vi "AIM664 Receive Continuous Capture.vi"() -> ()   [LabVIEW 2020]
uses:
  AIM664LV.lvlib
panel:
  out "QueueIdOut 2":u32
  out "GlobMonSize 2":u32=2153143691
  out "QueueIdOut":u32
  out "GlobMonSize":u32=2153143691
  in  "Strobe":u32(ring) items=["FDX_MON_STROBE_DIS", "FDX_MON_STROBE_STOP", "FDX_MON_STROBE_START"]
  in  "TriggerPosition":u32
  in  "CaptureMode":u32(ring)=1 items=["FDX_MON_SINGLE ", "FDX_MON_CONTINUOUS", "FDX_MON_SELECTIVE", "FDX_MON_RECORDING", "FDX_MON_REROS", "FDX_MON_HMU"]
  out "QueueStatus":T1 {"QueueStatus" items=["FDX_MON_STAT_EMPTY", "FDX_MON_STAT_ FILLED", "FDX_MON_STAT_ FULL", "FDX_MON_STAT_ OVERFLOW", "FDX_MON_STAT_ ERROR"]}
  out "GlobalStat Out":T2
  in  "Control":u32(ring) items=["FDX_RX_GS_RES_NO_CNT", "FDX_RX_GS_RES_ALL_CNT", "FDX_RX_GS_RES_ERR_CNT"]
  in  "PortMap":u32=1
  out "PortInitOut":T3 {"PortConfig" items=["FDX_SINGLE", "FDX_REDUNDANT"]}
  out "ResourceInfo 2":T4 {"PortMode" items=[" FDX_SINGLE", "FDX_REDUNDANT"]}
  out "ResourceInfo":T4 {"PortMode" items=[" FDX_SINGLE", "FDX_REDUNDANT"]}
  in  "Input Cluster 2":T5={"QueueCtrl"=1, "QueueId"=0, "RecordingFileName"="", "MaxFileSize"=0} {"QueueCtrl" items=["FDX_MON_QUEUE_CREATE", "FDX_MON_QUEUE_DELETE"]}
  in  "Stopp":bool
  out "Output Cluste":T6={"EntryRead"=0, "BytesRead"=0, "Synchronized"=0, "ReadBuffer"=[0, 0, 0, 0, 0, 0, 0, 0, 0, 0, 0, 0, 0, 0, 0, 0, 60, 0, 0, 0, 64, 64, 0, 48, 84, 0, 128, 0, 104, 8, 0, 0, 33, 75, 42, 162, 3, 0, 0, 0, 0, 60, 2, 0, 0, 1, 33, 32, 8, 0, 69, 0, 0, 45, 0, 0, 64, 0, 1, 17, 109, 162, 10, 1, 33, 1, 224, 224, 0, 60, 0, 24, 0, 23, 0, 25, 0, 0, 65, 66, 67, 68, 69, 70, 71, 72, 73, 74, 75, 76, 77, 78, 79, 80, 81, 84, 0, 5, 0, 5, 0, 5, 0, 5, 0, 5, 0, 5, 0, 5, 0, 5, 0, 5, 0, 5, 0, 5, 0, 5, 0, 5, 0, 5, 0, 5, 0, 5, 0, 0, 0, 0, 0, 0, 0, 0, 0, 0, 0, 0, 0, 0, 0, 0, 0, 0, 0, 0, 0, 0, 0, 0, 0, 0, 0, 0, 0, 0, 0, 0, 0, 0, 0, 0, 0, 0, 0, 0, 0, 0, 0, 0, 0, 0, 0, 0, 0, 0, 0, 0, 0, 0, 0, 0, 0, 0, 0, 0, 0, 0, 0, 0, 0, 0, 0, 0, 0, 0, 0, 0, 0, 0, 0, 0, 0, 0, 0, 0, 0, 0, 0, 0, 0, 0, 0, 0, 0, 0, 0, 0, 0, 0, 0, 0, 0, 0, 0, 0, 0, 0, 0, 0, 0, 0, 0, 0, 0, 0, 0, 0, 0, 0, 0, 0, 0, 0, 0, 0, 0, 0, 0, 0, 0, 0, 0, 0, 0, 0, 0, 0, 0, 0, 0, 0, 0, 0, 0, 0, 0, 0, 0, 0, 0, 0, 0, 0, 0, 0, 0, 0, 0, 0, 0, 0, 0, 0, 0, 0, 0, 0, 0, 0, 0, 0, 0, 0, 0, 0, 0, 0, 0, 0, 0, 0, 0, 0, 0, 0, 0, 0, 0, 0, 0, 0, 0, 0, 0, 0, 0, 0, 0, 0, 0, 0, 0, 0, 0, 0, 0, 0, 0, 0, 0, 0, 0, 0, 0, 0, 0, 0, 0, 0, 0, 0, 0, 0, 0, 0, 0, 0, 0, 0, 0, 0, 0, 0, 0, 0, 0, 0, 0, 0, 0, 0, 0, 0, 0, 0, 0, 0, 0, 0, 0, 0, 0, 0, 0, 0, 0, 0, 0, 0, 0, 0, 0, 0, 0, 0, 0, 0, 0, 0, 0, 0, 0, 0, 0, 0, 0, 0, 0, 0, 0, 0, 0, 0, 0, 0, 0, 0, 0, 0, 0, 0, 0, 0, 0, 0, 0, 0, 0, 0, 0, 0, 0, 0, 0, 0, 0, 0, 0, 0, 0, 0, 0, 0, 0, 0, 0, 0, 0, 0, 0, 0, 0, 0, 0, 0, 0, 0, 0, 0, 0, 0, 0, 0, 0, 0, 0, 0, 0, 0, 0, 0, 0, 0, 0, 0, 0, 0, 0, 0, 0, 0, 0, 0, 0, 0, 0, 0, 0, 0, 0, 0, 0, 0, 0, 0, 0, 0, 0, 0, 0, 0, 0, 0, 0, 0, 0, 0, 0, 0, 0, 0, 0, 0, 0, 0, 0, 0, 0, 0, 0, 0, 0, 0, 0, 0, 0, 0, 0, 0, 0, 0, 0, 0, 0, 0, 0, 0, 0, 0, 0, 0, 0, 0, 0, 0, 0, 0, 0, 0, 0, 0, 0, 0, 0, 0, 0, 0, 0, 0, 0, 0, 0, 0, 0, 0, 0, 0, 0, 0, 0, 0, 0, 0, 0, 0, 0, 0, 0, 0, 0, 0, 0, 0, 0, 0, 0, 0, 0, 0, 0, 0, 0, 0, 0, 0, 0, 0, 0, 0, 0, 0, 0, 0, 0, 0, 0, 0, 0, 0, 0, 0, 0, 0, 0, 0, 0, 0, 0, 0, 0, 0, 0, 0, 0, 0, 0, 0, 0, 0, 0, 0, 0, 0, 0, 0, 0, 0, 0, 0, 0, 0, 0, 0, 0, 0, 0, 0, 0, 0, 0, 0, 0, 0, 0, 0, 0, 0, 0, 0, 0, 0, 0, 0, 0, 0, 0, 0, 0, 0, 0, 0, 0, 0, 0, 0, 0, 0, 0, 0, 0, 0, 0, 0, 0, 0, 0, 0, 0, 0, 0, 0, 0, 0, 0, 0, 0, 0, 0, 0, 0, 0, 0, 0, 0, 0, 0, 0, 0, 0, 0, 0, 0, 0, 0, 0, 0, 0, 0, 0, 0, 0, 0, 0, 0, 0, 0, 0, 0, 0, 0, 0, 0, 0, 0, 0, 0, 0, 0, 0, 0, 0, 0, 0, 0, 0, 0, 0, 0, 0, 0, 0, 0, 0, 0, 0, 0, 0, 0, 0, 0, 0, 0, 0, 0, 0, 0, 0, 0, 0, 0, 0, 0, 0, 0, 0, 0, 0, 0, 0, 0, 0, 0, 0, 0, 0, 0, 0, 0, 0, 0, 0, 0, 0, 0, 0, 0, 0, 0, 0, 0, 0, 0, 0, 0, 0, 0, 0, 0, 0, 0, 0, 0, 0, 0, 0, 0, 0, 0, 0, 0, 0, 0, 0, 0, 0, 0, 0, 0, 0, 0, 0, 0, 0, 0, 0, 0, 0, 0, 0, 0, 0, 0, 0, 0, 0, 0, 0, 0, 0, 0, 0, 0, 0, 0, 0, 0, 0, 0, 0, 0, 0, 0, 0, 0, 0, 0, 0, 0, 0, 0, 0, 0, 0, 0, 0, 0, 0, 0, 0, 0, 0, 0, 0, 0, 0, 0, 0, 0, 0, 0, 0, 0, 0, 0, 0, 0, 0, 0, 0, 0, 0, 0, 0, 0, 0, 0, 0, 0, 0, 0, 0, 0, 0, 0, 0, 0, 0, 0, 0, 0, 0, 0, 0, 0, 0, 0, 0, 0, 0, 0, 0, 0, 0, 0, 0, 0, 0, 0, 0, 0, 0, 0, 0, 0, 0, 0, 0, 0, 0, 0, 0, 0, 0, 0, 0, 0, 0, 0, 0, 0, 0, 0, 0, 0, 0, 0, 0, 0, 0, 0, 0, 0, 0, 0, 0, 0, 0, 0, 0, 0, 0, 0, 0, 0, 0, 0, 0, 0, 0, 0, 0, 0, 0, 0, 0, 0, 0, 0, 0, 0, 0, 0, 0, 0, 0, 0, 0, 0, 0, 0, 0, 0, 0, 0, 0, 0, 0, 0, 0, 0, 0, 0, 0, 0, 0, 0, 0, 0, 0, 0, 0, 0, 0, 0, 0, 0, 0, 0, 0, 0, 0, 0, 0, 0, 0, 0, 0, 0, 0, 0, 0, 0, 0, 0, 0, 0, 0, 0, 0, 0, 0, 0, 0, 0, 0, 0, 0, 0, 0, 0, 0, 0, 0, 0, 0, 0, 0, 0, 0, 0, 0, 0, 0, 0, 0, 0, 0, 0, 0, 0, 0, 0, 0, 0, 0, 0, 0, 0, 0, 0, 0, 0, 0, 0, 0, 0, 0, 0, 0, 0, 0, 0, 0, 0, 0, 0, 0, 0, 0, 0, 0, 0, 0, 0, 0, 0, 0, 0, 0, 0, 0, 0, 0, 0, 0, 0, 0, 0, 0, 0, 0, 0, 0, 0, 0, 0, 0, 0, 0, 0, 0, 0, 0, 0, 0, 0, 0, 0, 0, 0, 0, 0, 0, 0, 0, 0, 0, 0, 0, 0, 0, 0, 0, 0, 0, 0, 0, 0, 0, 0, 0, 0, 0, 0, 0, 0, 0, 0, 0, 0, 0, 0, 0, 0, 0, 0, 0, 0, 0, 0, 0, 0, 0, 0, 0, 0, 0, 0, 0, 0, 0, 0, 0, 0, 0, 0, 0, 0, 0, 0, 0, 0, 0, 0, 0, 0, 0, 0, 0, 0, 0, 0, 0, 0, 0, 0, 0, 0, 0, 0, 0, 0, 0, 0, 0, 0, 0, 0, 0, 0, 0, 0, 0, 0, 0, 0, 0, 0, 0, 0, 0, 0, 0, 0, 0, 0, 0, 0, 0, 0, 0, 0, 0, 0, 0, 0, 0, 0, 0, 0, 0, 0, 0, 0, 0, 0, 0, 0, 0, 0, 0, 0, 0, 0, 0, 0, 0, 0, 0, 0, 0, 0, 0, 0, 0, 0, 0, 0, 0, 0, 0, 0, 0, 0, 0, 0, 0, 0, 0, 0, 0, 0, 0, 0, 0, 0, 0, 0, 0, 0, 0, 0, 0, 0, 0, 0, 0, 0, 0, 0, 0, 0, 0, 0, 0, 0, 0, 0, 0, 0, 0, 0, 0, 0, 0, 0, 0, 0, 0, 0, 0, 0, 0, 0, 0, 0, 0, 0, 0, 0, 0, 0, 0, 0, 0, 0, 0, 0, 0, 0, 0, 0, 0, 0, 0, 0, 0, 0, 0, 0, 0, 0, 0, 0, 0, 0, 0, 0, 0, 0, 0, 0, 0, 0, 0, 0, 0, 0, 0, 0, 0, 0, 0, 0, 0, 0, 0, 0, 0, 0, 0, 0, 0, 0, 0, 0, 0, 0, 0, 0, 0, 0, 0, 0, 0, 0, 0, 0, 0, 0, 0, 0, 0, 0, 0, 0, 0, 0, 0, 0, 0, 0, 0, 0, 0, 0, 0, 0, 0, 0, 0, 0, 0, 0, 0, 0, 0, 0, 0, 0, 0, 0, 0, 0, 0, 0, 0, 0, 0, 0, 0, 0, 0, 0, 0, 0, 0, 0, 0, 0, 0, 0, 0, 0, 0, 0, 0, 0, 0, 0, 0, 0, 0, 0, 0, 0, 0, 0, 0, 0, 0, 0, 0, 0, 0, 0, 0, 0, 0, 0, 0, 0, 0, 0, 0, 0, 0, 0, 0, 0, 0, 0, 0, 0, 0, 0, 0, 0, 0, 0, 0, 0, 0, 0, 0, 0, 0, 0, 0, 0, 0, 0, 0, 0, 0, 0, 0, 0, 0, 0, 0, 0, 0, 0, 0, 0, 0, 0, 0, 0, 0, 0, 0, 0, 0, 0, 0, 0, 0, 0, 0, 0, 0, 0, 0, 0, 0, 0, 0, 0, 0, 0, 0, 0, 0, 0, 0, 0, 0, 0, 0, 0, 0, 0, 0, 0, 0]} {"ReadBuffer" format="%x"}
  in  "Input Cluster":T7={"QueueId"=0, "EntryCount"=1, "ReadQualifier"=0, "MaxReadBytes"=1600} {"ReadQualifier" items=["FDX_MON_READ_FULL", "FDX_MON_READ_HEADER", "FDX_MON_READ_DATA"]}
  in  "Input Cluster":T5 {"QueueCtrl" items=["FDX_MON_QUEUE_CREATE", "FDX_MON_QUEUE_DELETE"]}
  in  "Input Cluster":T8={"ReceiveMode"=0, "DefaultPayloadMode"=0, "DefaultCronoMode"=1, "GlbMonBufferSizeIn"=0, "RerosDefaultOutputPortmap"=0} {"DefaultCronoMode" items=["cFDX_RX_DEFAULT_ENA_CNT", "FDX_RX_DEFAULT_MON_ENA_ALL", "FDX_RX_DEFAULT_MON_ENA_GOOD"]; "DefaultPayloadMode" items=["FDX_PAYLOAD_FULL", "FDX_PAYLOAD_IP_EXT", "FDX_PAYLOAD_IP", "FDX_PAYLOAD_MAC"]; "ReceiveMode" items=["FDX_RX_CHRONO", "FDX_RX_VL"]}
  out "GlbMonBufferSizeOut":u32
  in  "Input Cluster":T9={"SrvName"="local", "ClHostName"="local", "ClUser"="Brett", "ClApplication"="Test", "ClApplicationVersion"="V01.00", "ResourceID"=2, "Privileges"=4294967295} {"Privileges" items=["PRIVILEGES_ADMIN"=4294967295]}
  in  "Input Cluster":T9={"SrvName"="local", "ClHostName"="local", "ClUser"="Brett", "ClApplication"="Test", "ClApplicationVersion"="V01.00", "ResourceID"=1, "Privileges"=4294967295} {"Privileges" items=["PRIVILEGES_ADMIN"=4294967295]}
  in  "Input Cluster":T10={"SrvName"="local", "ResourceID"=1, "ResourceType"=0} {"ResourceType" items=["Board", "Port"]}
  out "Output Cluster 2":T11={"ResourceID"=0, "ResourceType"=0, "ResourceInfo"="0", "StructId"=0}
  in  "ServerRElement":u32=1
  in  "Input Cluster":T10={"SrvName"="local", "ResourceID"=2, "ResourceType"=1} {"ResourceType" items=["Board", "Port"]}
  out "Output Cluster":T11={"ResourceID"=0, "ResourceType"=0, "ResourceInfo"="0", "StructId"=0}
  in  "ServerRElement":u32=2
  out "NuOfResources":u32
  in  "SrvName":string="local"
  out "NuOfServers":u32=1
  # "ARINC 664 Receive Continuous Capture"
  # "Overview: Configure the board for Continuous Capture.\nRequirement: At least one AIM ARINC-664 board with installed AIM ARINC 664 BSP.\nRestrictions: None.\nInstruction:\n1. Run the VI.\n2. Verify the results in the indicators."
  # "Rx Port"
  # "Board"
  # "Rx Port"
  # "Board"
  # "FdxInitCvi"
  # "FdxLogoutCvi"
  # "CountServerResourcesCvi"
  # "GetServerResourcesCvi"
  # "QueryServerResourceCvi"
  # "FdxLoginCvi"
  # "FdxLogoutCvi"
  # "GetServerResourcesCvi"
  # "QueryServerResourceCvi"
  # "FdxRxModeControlCvi"
  # "FdxRxMonCaptureControlCvi"
  # "FdxLoginCvi"
  # "FdxCmdMonQueueControl"
  # "FdxRxControlCvi"
  # "FdxCmdMonQueueControl"
  # "FdxCmdRxPortInitCvi"
  # "FdxMonQueueStatusCvi"
  # "FdxCmdMonQueueReadCvi"
  # "FdxCmdRxGlblStatCvi"
  # "FdxRxControlCvi"
  # "Input"
  # "Input"
  # "Input"
  # "Input"
  # "Input"
  # "Input"
  # "Input"
  # "Input"
  # "Input"
  # "Output"
  # "Input"
  # "Input"
  # "Input"
  # "Input"
  # "Input"
  # "Input"
  # "Output"
  # "Output"
  # "Output"
  # "Output"
  # "Output"
  # "Output"
  # "Output"
  # "Output"
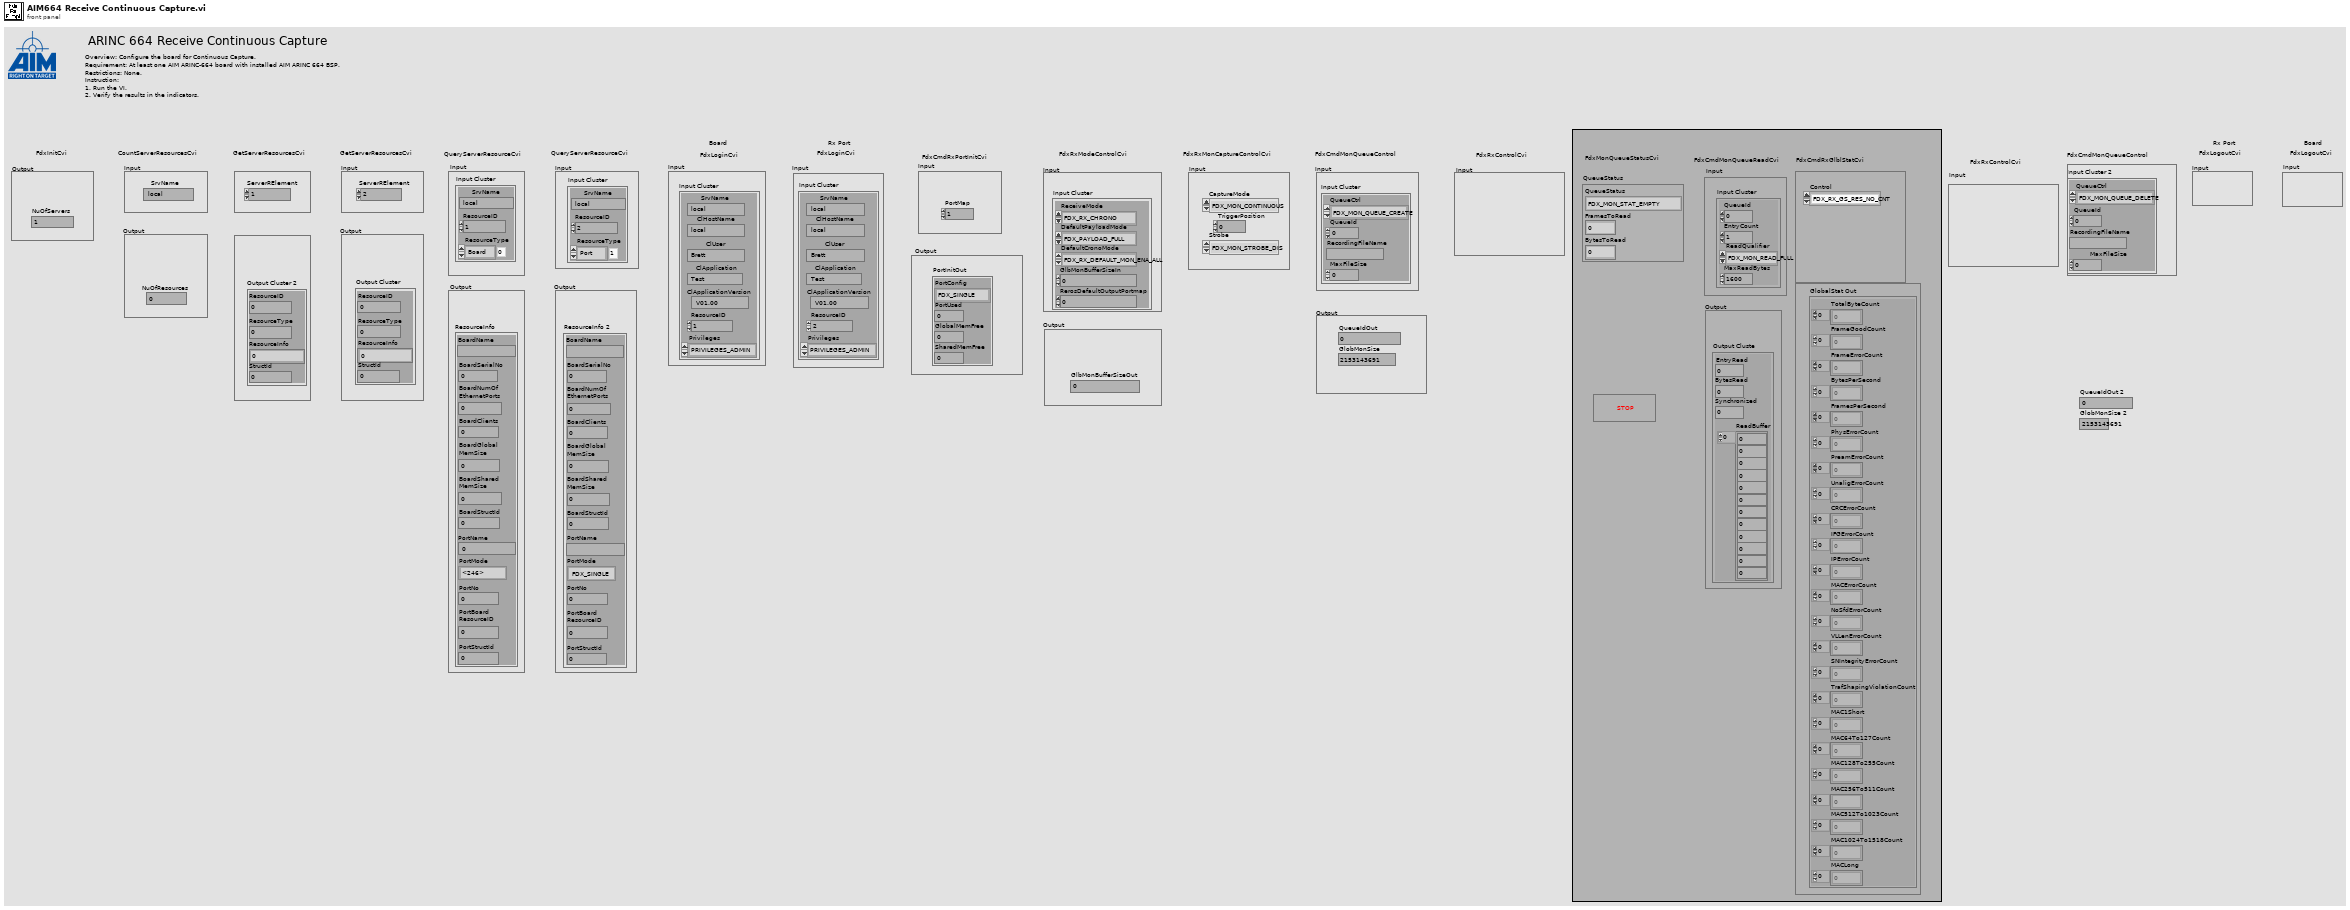
[diagram p1: front panel]
types:
  T1 = cluster{"QueueStatus":u32, "FramesToRead":u32, "BytesToRead":u32}
  T2 = cluster{"TotalByteCount":u32[], "FrameGoodCount":u32[], "FrameErrorCount":u32[], "BytesPerSecond":u32[], "FramesPerSecond":u32[], "PhysErrorCount":u32[], "PreamErrorCount":u32[], "UnaligErrorCount":u32[], "CRCErrorCount":u32[], "IFGErrorCount":u32[], "IPErrorCount":u32[], "MACErrorCount":u32[], "NoSfdErrorCount":u32[], "VLLenErrorCount":u32[], "SNIntegrityErrorCount":u32[], "TrafShapingViolationCount":u32[], "MAC1Short":u32[], "MAC64To127Count":u32[], "MAC128To255Count":u32[], "MAC256To511Count":u32[], "MAC512To1023Count":u32[], "MAC1024To1518Count":u32[], "MACLong":u32[]}
  T3 = cluster{"PortConfig":u32, "PortUsed":u32, "GlobalMemFree":u32, "SharedMemFree":u32}
  T4 = cluster{"BoardName":string, "BoardSerialNo":u32, "BoardNumOf\nEthernetPorts":u32, "BoardClients":u32, "BoardGlobal\nMemSize":u32, "BoardShared\nMemSize":u32, "BoardStructId":u32, "PortName":string, "PortMode":u32, "PortNo":u32, "PortBoard\nResourceID":u32, "PortStructId":u32}
  T5 = cluster{"QueueCtrl":u32, "QueueId":u32, "RecordingFileName":string, "MaxFileSize":u32}
  T6 = cluster{"EntryRead":u32, "BytesRead":u32, "Synchronized":u32, "ReadBuffer":u8[]}
  T7 = cluster{"QueueId":u32, "EntryCount":u32, "ReadQualifier":u32, "MaxReadBytes":u32}
  T8 = cluster{"ReceiveMode":u32, "DefaultPayloadMode":u32, "DefaultCronoMode":u32, "GlbMonBufferSizeIn":u32, "RerosDefaultOutputPortmap":u32}
  T9 = cluster{"SrvName":string, "ClHostName":string, "ClUser":string, "ClApplication":string, "ClApplicationVersion":string, "ResourceID":u32, "Privileges":u32}
  T10 = cluster{"SrvName":string, "ResourceID":u32, "ResourceType":u32}
  T11 = cluster{"ResourceID":u32, "ResourceType":u32, "ResourceInfo":string, "StructId":u32}
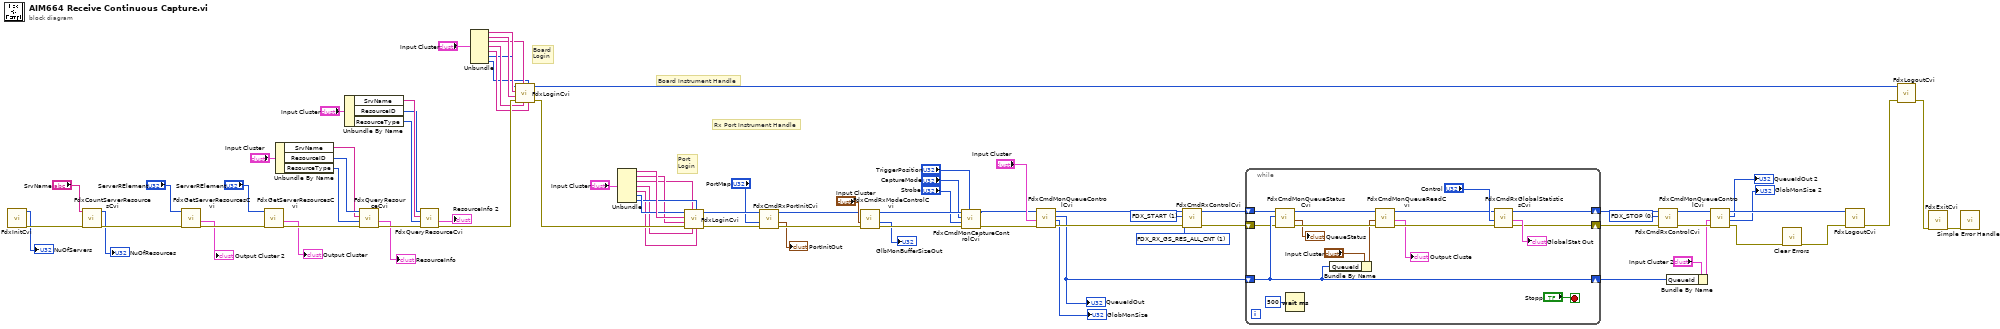
[diagram p0: block diagram]
diagram:
  w4 = u32 0 items=["FDX_STOP", "FDX_START"] ("StartMode")
  w5 = u32 1 items=["FDX_RX_GS_RES_NO_CNT", "FDX_RX_GS_RES_ALL_CNT", "FDX_RX_GS_RES_ERR_CNT "] ("GlobalStatisticReset")
  w6 = u32 1 items=["FDX_STOP", "FDX_START"] ("StartMode")
  # "Rx Port Instrument Handle"
  # "Port\nLogin"
  # "Board Instrument Handle"
  # "Board\nLogin"
  n1 = call "FdxInitCvi.vi"() -> ("error out"=w80:errorcluster, "Number of Servers"=→"NuOfServers":u32)  [unwired: 10 in]
  n2 = call "FdxCountServerResourcesCvi.vi"("error in"=w80, "SrvName (local)"="SrvName") -> ("error out"=w79:errorcluster, "Number of Resources"=→"NuOfResources":u32)  [unwired: 8 in]
  n3 = call "FdxGetServerResourcesCvi.vi"("error in"=w79, "ServerRElement"="ServerRElement") -> ("error out"=w78:errorcluster, "ServerResourceInfo"=→"Output Cluster 2":T11)  [unwired: 4 in, 4 out]
  n4 = call "FdxGetServerResourcesCvi.vi"("error in"=w78, "ServerRElement"="ServerRElement") -> ("error out"=w81:errorcluster, "ServerResourceInfo"=→"Output Cluster":T11)  [unwired: 4 in, 4 out]
  n5 = Unbundle By Name("Input Cluster") -> ("SrvName"=w44:string, "ResourceID"=w46:u32, "ResourceType"=w45:u32)
  n6 = Unbundle By Name("Input Cluster") -> ("SrvName"=w42:string, "ResourceID"=w41:u32, "ResourceType"=w40:u32)
  n7 = call "FdxQueryResourceCvi.vi"("error in"=w81, "ResourceType"=w45, "SrvName"=w44, "ResourceID"=w46) -> ("error out"=w77:errorcluster, "ResourceInfo"=→"ResourceInfo":T4)  [unwired: 5 in, 1 out]
  n8 = call "FdxQueryResourceCvi.vi"("error in"=w77, "ResourceType"=w40, "SrvName"=w42, "ResourceID"=w41) -> ("error out"=w76:errorcluster, "ResourceInfo"=→"ResourceInfo 2":T4)  [unwired: 5 in, 1 out]
  n9 = Unbundle("Input Cluster") -> ("SrvName"=w38:string, "ClHostName"=w37:string, "ClUser"=w33:string, "ClApplication"=w36:string, "ClApplicationVersion"=w35:string, "ResourceID"=w34:u32, "Privileges"=w32:u32)
  n10 = call "FdxLoginCvi.vi"("ClApplicationVersion"=w35, "Privileges"=w32, "ClApplication"=w36, "ClUser"=w33, "error in"=w76, "ClHostName"=w37, "SrvName"=w38, "ResourceID"=w34) -> ("error out"=w71:errorcluster, "InstrumentHandle"=w62:u32)  [unwired: 2 in]
  n11 = Unbundle("Input Cluster") -> ("SrvName"=w30:string, "ClHostName"=w25:string, "ClUser"=w24:string, "ClApplication"=w27:string, "ClApplicationVersion"=w26:string, "ResourceID"=w29:u32, "Privileges"=w28:u32)
  n12 = call "FdxLoginCvi.vi"("ClApplicationVersion"=w26, "Privileges"=w28, "ClApplication"=w27, "ClUser"=w24, "error in"=w71, "ClHostName"=w25, "SrvName"=w30, "ResourceID"=w29) -> ("error out"=w68:errorcluster, "InstrumentHandle"=w53:u32)  [unwired: 2 in]
  n13 = call "FdxCmdRxPortInitCvi.vi"("error in"=w68, "PortMap"="PortMap", "InstrumentHandle_port"=w53) -> ("error out"=w67:errorcluster, "PortInitOut"=→"PortInitOut":T3, "InstrumentHandle_port"=w23:u32)  [unwired: 6 in]
  n14 = call "FdxCmdRxModeControlCvi.vi"("error in"=w67, "RxModeControlIn"="Input Cluster", "InstrumentHandle_port"=w23) -> ("error out"=w75:errorcluster, "GlbMonBufferSizeOut"=→"GlbMonBufferSizeOut":u32, "InstrumentHandle_port"=w22:u32)  [unwired: 6 in]
  n15 = call "FdxCmdMonCaptureControlCvi.vi"("TriggerPosition"="TriggerPosition", "error in"=w75, "Strobe"="Strobe", "CaptureMode"="CaptureMode", "InstrumentHandle_port"=w22) -> ("error out"=w74:errorcluster, "InstrumentHandle_port"=w21:u32)  [unwired: 5 in]
  n16 = call "FdxCmdMonQueueControlCvi.vi"("error in"=w74, "Q Ctrl In"="Input Cluster", "InstrumentHandle_port"=w21) -> ("error out"=w73:errorcluster, "GlobMonSize"=→"GlobMonSize":u32, "QueueIdOut"=w8:u32, "InstrumentHandle_port"=w20:u32)  [unwired: 5 in]
  "QueueIdOut" <- w8
  n17 = call "FdxCmdRxControlCvi.vi"("error in"=w73, "GlobalStatisticReset"=w5, "StartMode"=w6, "InstrumentHandle_port"=w20) -> ("error out"=w17:errorcluster, "InstrumentHandle_port"=w19:u32)  [unwired: 6 in]
  n18 = while {
    shift-right: [w84] -> w18
    shift-left: w19 -> [w87]
    shift-right: [w82] -> w16
    shift-left: w17 -> [w83]
    shift-right: [w89] -> w55
    shift-left: w8 -> [w89]
    stop <- "Stopp" stop-if-true
    n19 = call "FdxCmdMonQueueStatusCvi.vi"("error in"=w83, "QueueId"=w89, "InstrumentHandle_port"=w87) -> ("error out"=w98:errorcluster, "QueueStatus"=→"QueueStatus":T1, "InstrumentHandle_port"=w86:u32)  [unwired: 6 in]
    n20 = Wait (ms)(milliseconds to wait=u32 500 ("Zu wartende ms")) -> ()  [unwired: 1 out]
    n21 = Bundle By Name(cluster="Input Cluster", "QueueId"=w89) -> (w94:T7)
    n22 = call "FdxCmdMonQueueReadCvi.vi"("error in"=w98, "QueueReadIn"=w94, "InstrumentHandle_port"=w86) -> ("error out"=w97:errorcluster, "QueueReadOut"=→"Output Cluste":T6, "InstrumentHandle_port"=w85:u32)  [unwired: 6 in]
    n23 = call "FdxCmdRxGlobalStatisticsCvi.vi"("error in"=w97, "Control"="Control", "InstrumentHandle_port"=w85) -> ("error out"=w82:errorcluster, "GlobalStat Out"=→"GlobalStat Out":T2, "InstrumentHandle_port"=w84:u32)  [unwired: 6 in]
  }
  n24 = call "FdxCmdRxControlCvi.vi"("error in"=w16, "StartMode"=w4, "InstrumentHandle_port"=w18) -> ("error out"=w70:errorcluster, "InstrumentHandle_port"=w15:u32)  [unwired: 7 in]
  n25 = Bundle By Name(cluster="Input Cluster 2", "QueueId"=w55) -> (w56:T5)
  n26 = call "FdxCmdMonQueueControlCvi.vi"("error in"=w70, "Q Ctrl In"=w56, "InstrumentHandle_port"=w15) -> ("error out"=w13:errorcluster, "GlobMonSize"=→"GlobMonSize 2":u32, "QueueIdOut"=→"QueueIdOut 2":u32, "InstrumentHandle_port"=w14:u32)  [unwired: 5 in]
  n27 = call <vilib>:"Clear Errors.vi"("error in (no error)"=w13) -> ("error out"=w12:errorcluster)  [unwired: 5 in, 1 out]
  n28 = call "FdxLogoutCvi.vi"("error in"=w12, "InstrumentHandle"=w14) -> ("error out"=w72:errorcluster)  [unwired: 9 in]
  n29 = call "FdxLogoutCvi.vi"("error in"=w72, "InstrumentHandle"=w62) -> ("error out"=w69:errorcluster)  [unwired: 9 in]
  n30 = call "FdxExitCvi.vi"("error in"=w69) -> ("error out"=w1:errorcluster)  [unwired: 10 in]
  n31 = call <vilib>:"Simple Error Handler.vi"("error in (no error)"=w1) -> ()  [unwired: 4 in, 5 out]
